vi "signal processingclass.vi"() -> ()   [LabVIEW 2023]
uses:
  <vilib>/express/express analysis/Spectral/Block/exnSpectralBlock spectral measurements power poly.vi
  <vilib>/express/express analysis/Spectral/Block/exnSpectralBlock spectral measurements power WFM.vi
  <vilib>/express/express analysis/Spectral/XNode/ExpressSpectralMeasurementsBlockNode.xnode
  <vilib>/measure/NI_MABase.lvlib
panel:
  in  "Lower Cut-Off":dbl=100.0
  out "Waveform Graph 3":dynamicdata(graph)
  out "Waveform Graph 2":cluster{"f0":dbl, "df":dbl, "magnitude":dbl[]}(graph)
  in  "stop":bool
  in  "offset 2":dbl format="%0.2p"
  in  "amplitude 2":dbl=1.0 format="%0.2p"
  in  "phase 2":dbl format="%.2p"
  in  "frequency 2":dbl=10.0 format="%0.2p"
  out "Waveform Graph":waveform(dbl)(graph)
  in  "frequency":dbl=10.0 format="%0.2p"
  in  "phase":dbl format="%.2p"
  in  "amplitude":dbl=1.0 format="%0.2p"
  in  "offset":dbl format="%0.2p"
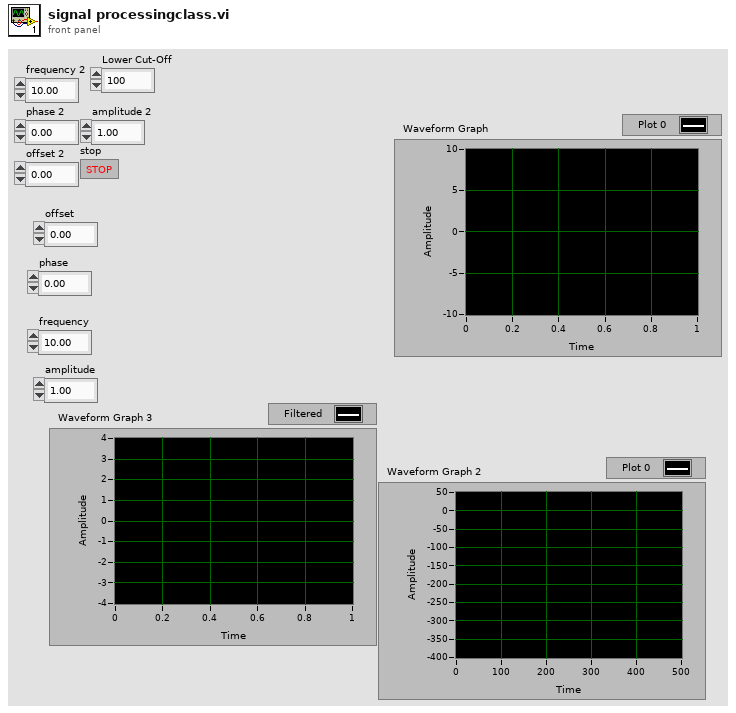
[diagram p1: front panel]
types:
  T1 = cluster{"averaging mode":u16, "weighting mode":u16, "number of averages":u32}
  T2 = cluster{"dB On (F)":bool, "unwrap phase (F)":bool, "convert to degree (F)":bool}
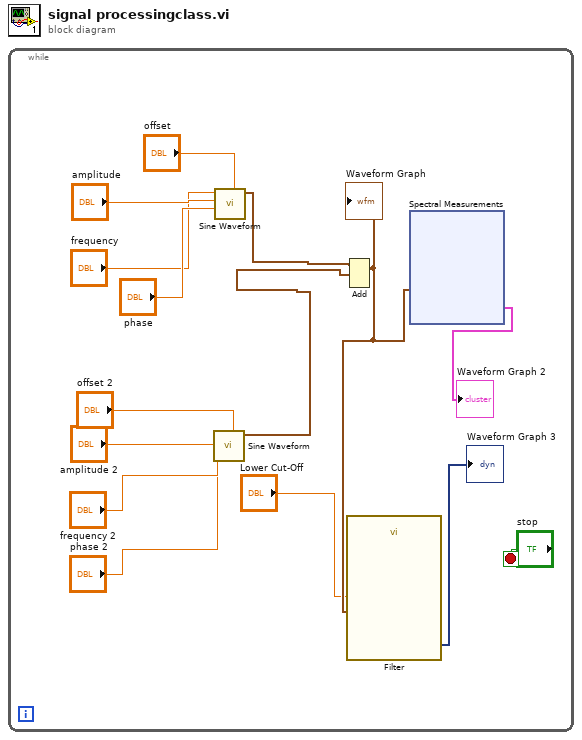
[diagram p0: block diagram]
diagram:
  n1 = while {
    stop <- "stop" stop-if-true
    n2 = call <vilib>:"Sine Waveform.vi"("offset"="offset 2", "phase"="phase 2", "amplitude"="amplitude 2", "frequency"="frequency 2") -> ("signal out"=w6:waveform(dbl))  [unwired: 6 in, 1 out]
    n3 = call <vilib>:"Sine Waveform.vi"("offset"="offset", "phase"="phase", "amplitude"="amplitude", "frequency"="frequency") -> ("signal out"=w7:waveform(dbl))  [unwired: 6 in, 1 out]
    n4 = Add(1:w6, 2:w7) -> (0:w4:waveform(dbl))  [unwired: 1 in, 1 out]
    "Waveform Graph" <- w4
    n5 = call "Filter"("Lower Cut-Off"="Lower Cut-Off", "Signal"=w4) -> ("Filtered Signal"=→"Waveform Graph 3":dynamicdata)  [unwired: 8 in, 1 out]
    n6 = xnode "Spectral Measurements"("Signals"=w4) -> ("Power Spectrum"=→"Waveform Graph 2":cluster{"f0":dbl, "df":dbl, "magnitude":dbl[]})  [unwired: 1 in, 1 out]
  }
